vi "SMP Example.vi"() -> ()   [LabVIEW 2013]
uses:
  SMP.lvclass
  Polymorphic VIs/AddOperationsAsPipe.vi
  Data types/operation.ctl
  Polymorphic VIs/AddSingleOperation.vi
panel:
  in  "Load (no pipe)":bool
  in  "Load (pipe)":bool
  in  "File path":path
  out "File contents as string":string
  out "error out":errorcluster
  out "stop":bool
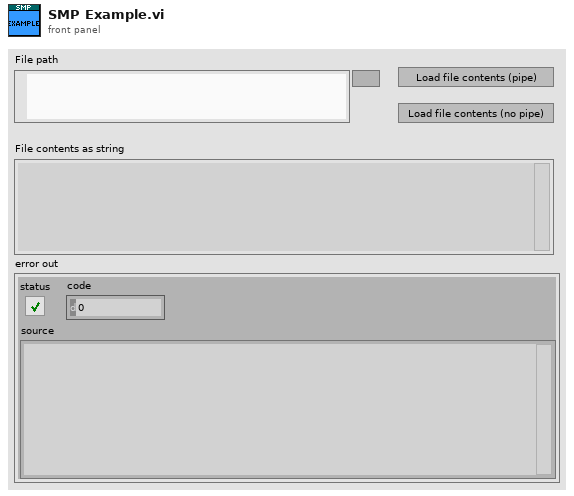
[diagram p1: front panel]
types:
  T1 = typedef "SMP.lvclass/operation.ctl" = cluster{"Name":string, "Data":variant}
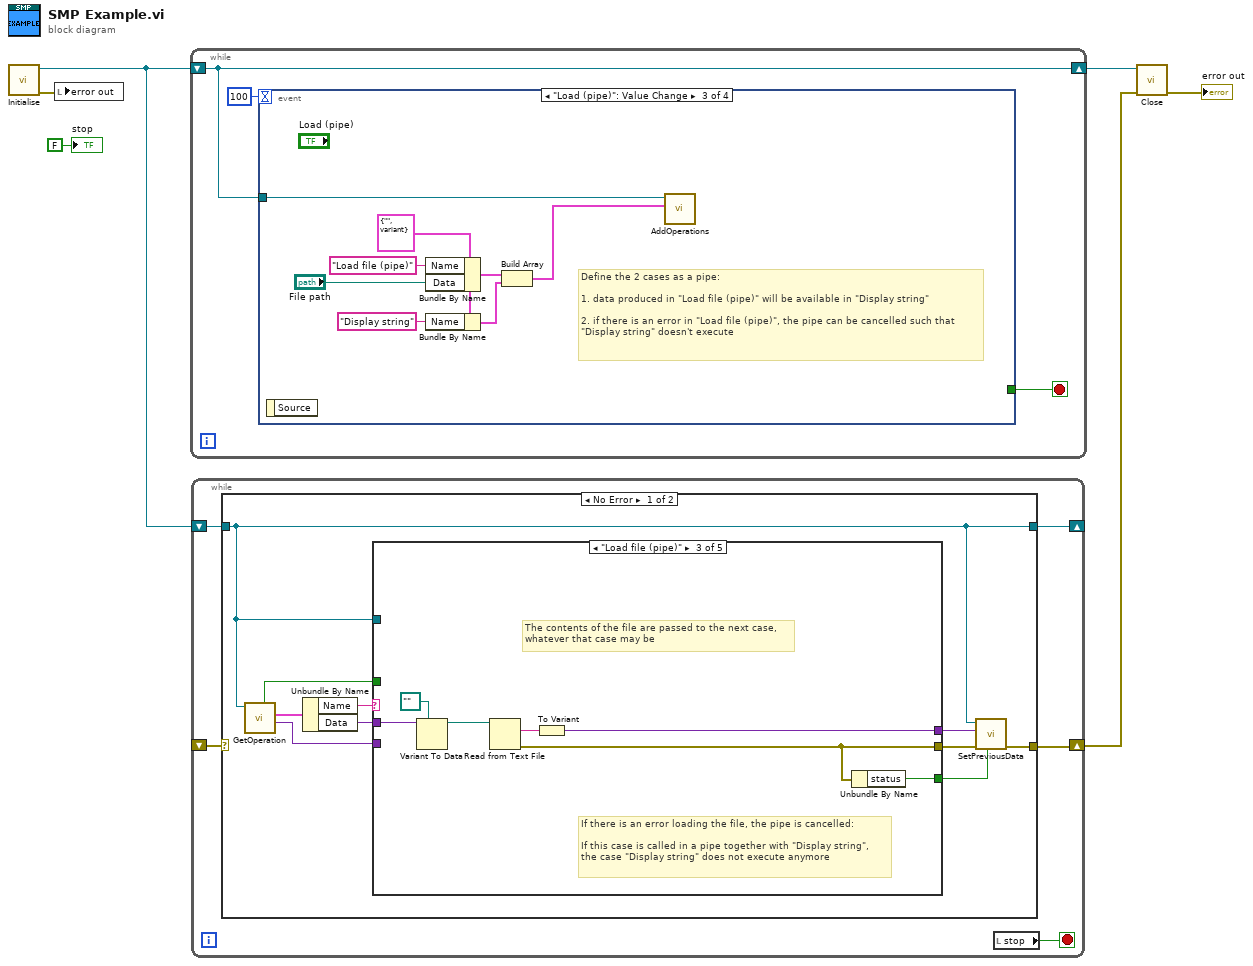
[diagram p0: block diagram]
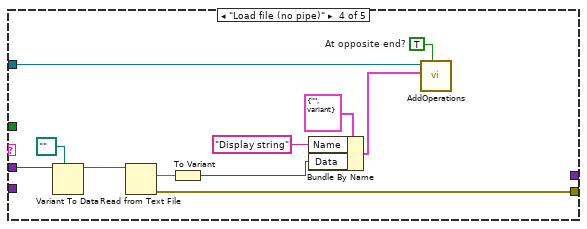
[diagram p4: hidden frame]
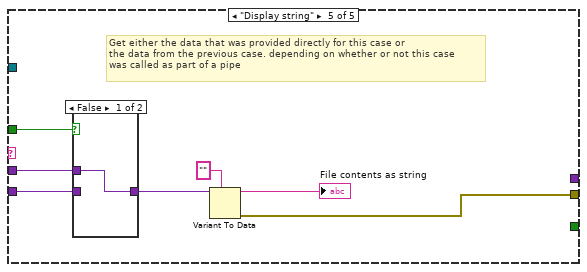
[diagram p5: hidden frame]
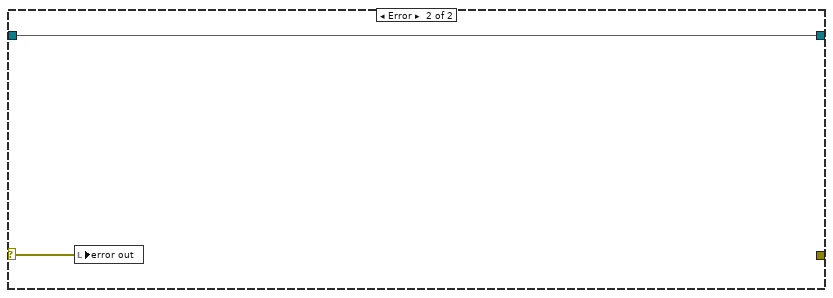
[diagram p7: hidden frame]
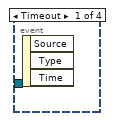
[diagram p8: hidden frame]
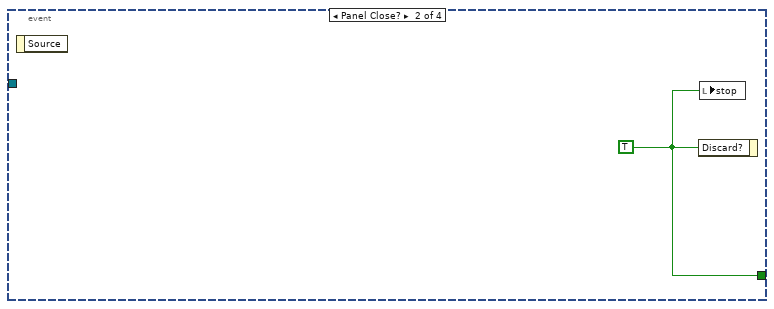
[diagram p9: hidden frame]
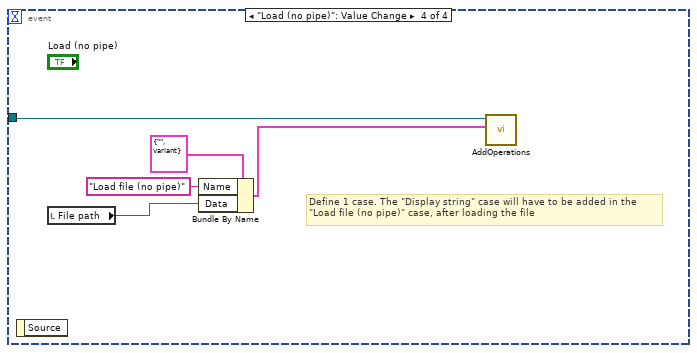
[diagram p10: hidden frame]
diagram:
  n1 = call "Initialise.vi"() -> ("error out"=w3:errorcluster, "SMP out"=w6:refnum<class "SMP.lvclass">)  [unwired: 10 in]
  n2 = local write "error out"(w3) -> ()
  n3 = while {
    shift-right: [w8] -> w5
    shift-left: w6 -> [w8]
    stop <- w7 stop-if-true
    n4 = event shown="[2] \"Load (pipe)\": Value Change" {
      selector: _ -> [_ _ _ _]
      dyn-events: _ -> [_ _ _ _]
      timeout: 100 -> [_ _ _ _]
      tunnel: w8 -> [_ _ w18 w19]
      tunnel: [_ w10 _ _] -> w7
      event Timeout {
        n5 = event-data() -> ()  [unwired: 1 in, 3 out]
      }
      event Panel Close? {
        w10 = TRUE ("Discard?")
        n6 = event-data() -> ()  [unwired: 1 in, 1 out]
        n7 = event-data("Discard?"=w10) -> ()  [unwired: 1 in, 1 out]
        n8 = local write "stop"(w10) -> ()
      }
      event "Load (pipe)": Value Change {
        w15 = T1 {"Name"="", "Data"=variant} ("Element")
        # "Define the 2 cases as a pipe:\n\n1. data produced in \"Load file (pipe)\" will be available in \"Display string\"\n\n2. if there is an error in \"Load file (pipe)\", the pipe can be cancelled such that\n\"Display string\" doesn't execute"
        n9 = event-data() -> ()  [unwired: 1 in, 1 out]
        n10 = Bundle By Name(cluster=w15, "Name"="Load file (pipe)", "Data"="File path") -> (w14:T1)
        n11 = Bundle By Name(cluster=w15, "Name"="Display string") -> (w13:T1)
        n12 = Build Array(w14, w13) -> (w12:T1[])
        n13 = call-poly "AddOperations.vi"("Operations"=w12, "SMP in"=w18) -> ()  [unwired: 8 in, 2 out]
      }
      event "Load (no pipe)": Value Change {
        # "Define 1 case. The \"Display string\" case will have to be added in the\n\"Load file (no pipe)\" case, after loading the file"
        n14 = event-data() -> ()  [unwired: 1 in, 1 out]
        n15 = local read "File path"() -> (w20:path)
        n16 = Bundle By Name(cluster=T1 {"Name"="", "Data"=variant} ("Element"), "Name"="Load file (no pipe)", "Data"=w20) -> (w21:T1)
        n17 = call-poly "AddOperations.vi"("Operation"=w21, "SMP in"=w19) -> ()  [unwired: 8 in, 2 out]
      }
    }
  }
  n18 = while {
    shift-right: [w26] -> _
    shift-left: w6 -> [w27]
    shift-right: [w25] -> w2
    shift-left: _ -> [w24]
    stop <- w28 stop-if-true
    n19 = case shown="No Error" w24 {
      selector: w24 -> [_ w67]
      tunnel: w27 -> [w30 w66]
      tunnel: [w30 w66] -> w26
      tunnel: [w38 _] -> w25
      frame No Error {
        n20 = call "GetOperation.vi"("SMP in"=w30) -> ("Previous data"=w36:variant, "Operation"=w37:T1, "Pipe operation?"=w29:bool)  [unwired: 5 in, 3 out]
        n21 = Unbundle By Name(w37) -> ("Name"=w35:string, "Data"=w34:variant)
        n22 = case shown="\"Load file (pipe)\"" w35 {
          tunnel: w36 -> [_ _ _ _ w59]
          tunnel: w34 -> [_ _ w45 w56 w58]
          tunnel: w29 -> [_ _ _ _ w61]
          tunnel: [_ _ w40 w52 w57] -> w33
          tunnel: [_ _ w41 _ _] -> w31
          tunnel: [_ _ w39 _ _] -> w32
          tunnel: w30 -> [_ _ _ w51 _]
          frame Default {
          }
          frame "" {
          }
          frame "Load file (pipe)" {
            # "The contents of the file are passed to the next case,\nwhatever that case may be"
            # "If there is an error loading the file, the pipe is cancelled:\n\nIf this case is called in a pipe together with \"Display string\",\nthe case \"Display string\" does not execute anymore"
            n23 = Variant To Data(type=path "" ("Path"), Variant=w45) -> (data=w43:path)  [unwired: 1 in, 1 out]
            n24 = Read from Text File(file (use dialog)=w43) -> (text=w42:string, error out=w40:errorcluster)  [unwired: 3 in, 2 out]
            n25 = To Variant(anything=w42) -> (Variant=w41:variant)
            n26 = Unbundle By Name(w40) -> ("status"=w39:bool)
          }
          frame "Load file (no pipe)" {
            w46 = TRUE  # At opposite end?
            n27 = Variant To Data(type=path "" ("Path"), Variant=w56) -> (data=w54:path)  [unwired: 1 in, 1 out]
            n28 = Read from Text File(file (use dialog)=w54) -> (text=w53:string, error out=w52:errorcluster)  [unwired: 3 in, 2 out]
            n29 = To Variant(anything=w53) -> (Variant=w49:variant)
            n30 = Bundle By Name(cluster=T1 {"Name"="", "Data"=variant} ("Element"), "Name"="Display string", "Data"=w49) -> (w47:T1)
            n31 = call-poly "AddOperations.vi"("At opposite end?"=w46, "Operation"=w47, "SMP in"=w51) -> ()  [unwired: 7 in, 2 out]
          }
          frame "Display string" {
            # "Get either the data that was provided directly for this case or\nthe data from the previous case. depending on whether or not this case\nwas called as part of a pipe"
            n32 = case shown="False" w61 {
              tunnel: [w64 w65] -> w60
              tunnel: w59 -> [_ w65]
              tunnel: w58 -> [w64 _]
              frame False {
              }
              frame True {
              }
            }
            n33 = Variant To Data(type="" ("Path"), Variant=w60) -> (data=→"File contents as string":string, error out=w57:errorcluster)  [unwired: 1 in]
          }
        }
        n34 = call "SetPreviousData.vi"("Cancel pipe? (F)"=w32, "error in (no error)"=w33, "Data"=w31, "SMP in"=w30) -> ("error out"=w38:errorcluster)  [unwired: 6 in, 1 out]
      }
      frame Error {
        n35 = local write "error out"(w67) -> ()
      }
    }
    n36 = local read "stop"() -> (w28:bool)
  }
  n37 = call "Close.vi"("error in (no error)"=w2, "SMP in"=w5) -> ("error out"=→"error out":errorcluster)  [unwired: 9 in]
  "stop" <- FALSE ("stop")
